vi "Close ActiveX Reference.vi"(8 "error in":errorcluster, 11 "IMG_SRC in":refnum<class "IMG_SRC.lvclass">) -> (0 "error out":errorcluster, 3 "IMG_SRC out":refnum<class "IMG_SRC.lvclass">)   [LabVIEW 2018, in "IMG_SRC.lvlib" / "IMG_SRC.lvclass"]
uses:
  IMG_SRC.lvclass
  IMG_SRC.lvclass/IMG_SRC.ctl
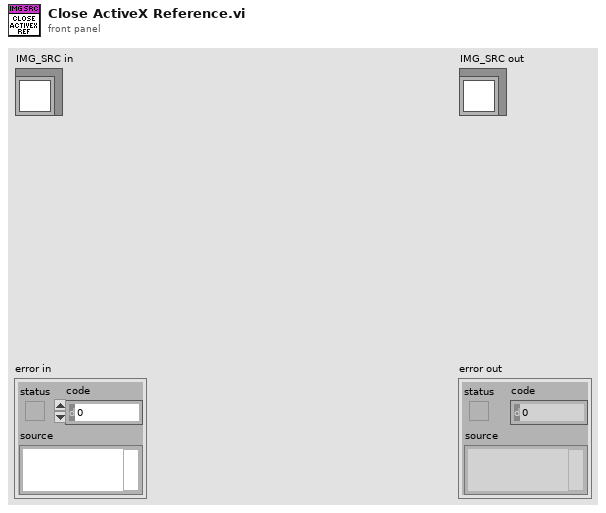
[diagram p1: front panel]
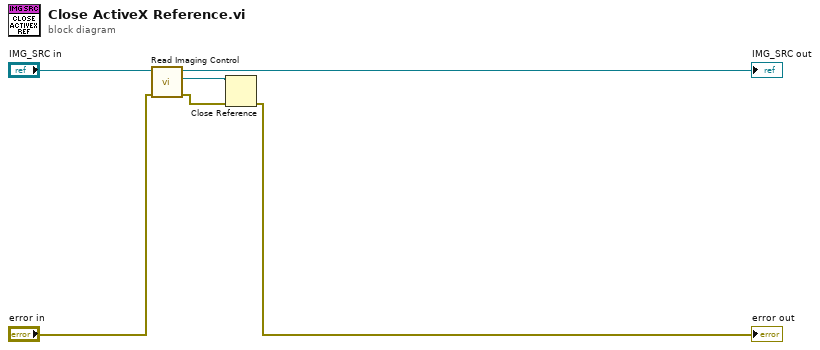
[diagram p0: block diagram]
diagram:
  n1 = call "Read Imaging Control.vi"("error in (no error)"="error in", "IMG_SRC in"="IMG_SRC in") -> ("error out"=w2:errorcluster, "Imaging Control"=w3:refnum<k7>, "IMG_SRC out"=→"IMG_SRC out":refnum<class "IMG_SRC.lvclass">)  [unwired: 7 in]
  n2 = Close Reference(reference=w3, error in (no error)=w2) -> (error out=→"error out":errorcluster)
